vi "VIV_VIPM Post Install Process.vi"(8 "Error In":errorcluster, 10 "Files Installed":path[](array[path]), 11 "Package Name":string) -> (0 "Error Out":errorcluster, 2 "Files Replaced":path[](array[path]), 3 "New Files Added":path[](array[path]))   [LabVIEW 2018]
uses:
  <vilib>/Utility/file.llb/Write Delimited Spreadsheet (string).vi
  <vilib>/zip/NI_Unzip.lvlib
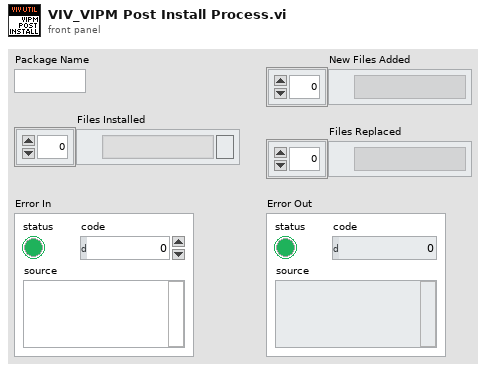
[diagram p1: front panel]
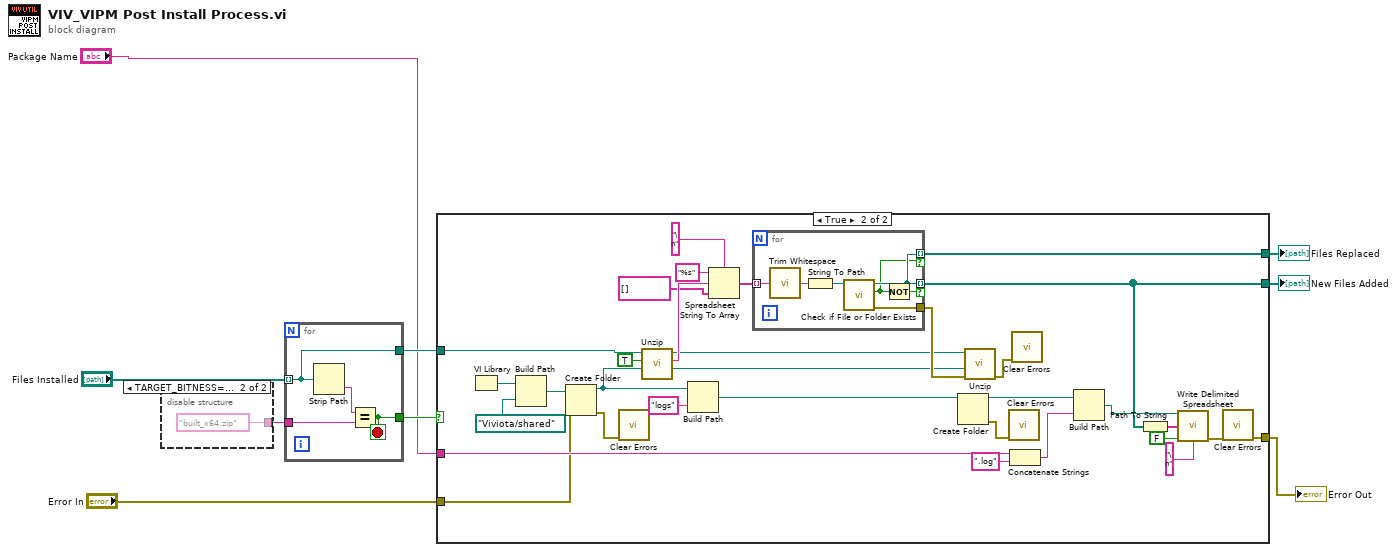
[diagram p0: block diagram]
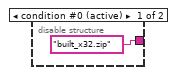
[diagram p2: hidden frame]
diagram:
  n1 = disable-structure shown="TARGET_BITNESS==64" {
    disable-tunnel: ["built_x32.zip" "built_x64.zip"] -> w7
    frame condition #0 (active) {
    }
    frame condition #1 {
    }
  }
  n2 = for {
    tunnel: w7 -> [w14]
    tunnel: "Files Installed" -> [w12] mode=indexing
    tunnel: [w13] -> w8
    tunnel: [w12] -> w9
    stop <- w13 stop-if-true
    n3 = Strip Path(path=w12) -> (name=w15:string)  [unwired: 1 out]
    n4 = Equal?(x=w15, y=w14) -> (x = y?=w13:bool)
  }
  n5 = case shown="True" w8 {
    tunnel: w9 -> [_ w22]
    tunnel: "Package Name" -> [_ w38]
    tunnel: [_ w20] -> w1
    tunnel: [_ w19] -> w4
    tunnel: [_ w18] -> w3
    tunnel: "Error In" -> [_ w16]
    frame False {
    }
    frame True {
      n6 = VI Library() -> (path=w45:path)
      n7 = Build Path(base path=w45, name or relative path=path "Viviota/shared") -> (appended path=w43:path)
      n8 = Create Folder(path (use dialog)=w43, error in=w16) -> (created path=w21:path, error out=w42:errorcluster)  [unwired: 1 in, 1 out]
      n9 = call <vilib>:"Clear Errors.vi"("error in (no error)"=w42) -> ()  [unwired: 5 in, 2 out]
      n10 = call <vilib>:"Unzip.vi"("Target directory (same as Zip file if empty)"=w21, "Preview only?"=TRUE, "Zip file"=w22) -> ("Preview"=w28:string)  [unwired: 6 in, 2 out]
      n11 = Build Path(base path=w21, name or relative path="logs") -> (appended path=w40:path)
      n12 = Spreadsheet String To Array(delimiter (Tab)="\n", format string="%s", spreadsheet string=w28, array type (2D Dbl)=string[] []) -> (array=w24:string[])
      n13 = for {
        tunnel: w24 -> [w52] mode=indexing
        tunnel: [w48] -> w19 mode=indexing if=w50
        tunnel: [w49] -> w23
        tunnel: [w48] -> w18 mode=indexing if=w47
        n14 = call <vilib>:"Trim Whitespace.vi"("string"=w52) -> ("trimmed string"=w46:string)  [unwired: 1 in]
        n15 = String To Path(string=w46) -> (path=w51:path)
        n16 = call <vilib>:"Check if File or Folder Exists.vi"("path"=w51) -> ("error out"=w49:errorcluster, "file or folder exists?"=w47:bool, "dup path"=w48:path)  [unwired: 8 in]
        n17 = Not(x=w47) -> (.not. x?=w50:bool)
      }
      n18 = Create Folder(path (use dialog)=w40) -> (created path=w35:path, error out=w39:errorcluster)  [unwired: 2 in, 1 out]
      n19 = call <vilib>:"Unzip.vi"("error in (no error)"=w23, "Target directory (same as Zip file if empty)"=w21, "Zip file"=w22) -> ("error out"=w17:errorcluster)  [unwired: 6 in, 2 out]
      n20 = call <vilib>:"Clear Errors.vi"("error in (no error)"=w39) -> ()  [unwired: 5 in, 2 out]
      n21 = Concatenate Strings(w38, ".log" ("string")) -> (w34:string)
      n22 = call <vilib>:"Clear Errors.vi"("error in (no error)"=w17) -> ()  [unwired: 5 in, 2 out]
      n23 = Build Path(base path=w35, name or relative path=w34) -> (appended path=w33:path)
      n24 = Path To String(path=w19) -> (string=w36:string[])
      n25 = call-poly <vilib>:"Write Delimited Spreadsheet.vi"("file path (dialog if empty)"=w33, "1D data"=w36, "append to file? (new file:F)"=FALSE, "delimiter (\\t)"="\n" ("delimiter (\\t)")) -> ("error out"=w31:errorcluster)  [unwired: 10 in, 1 out]
      n26 = call <vilib>:"Clear Errors.vi"("error in (no error)"=w31) -> ("error out"=w20:errorcluster)  [unwired: 5 in, 1 out]
    }
  }
  "New Files Added" <- w4
  "Files Replaced" <- w3
  "Error Out" <- w1
